vi "pcfs_main_fsm_loop.vi"(8 "error in (no error)":errorcluster, 11 "pcfs in":refnum<class "pcfs.lvclass">) -> (0 "error out":errorcluster, 3 "pcfs out":refnum<class "pcfs.lvclass">)   [LabVIEW 2015, in "pcfs.lvclass"]
uses:
  pcfs.lvclass
  pcfs.lvclass/pcfs.ctl
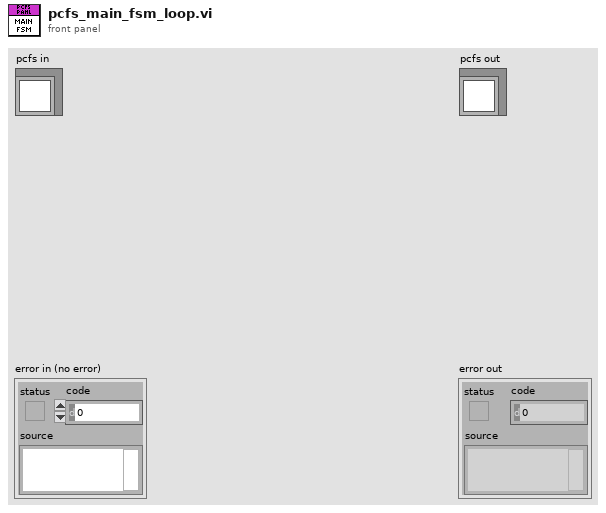
[diagram p1: front panel]
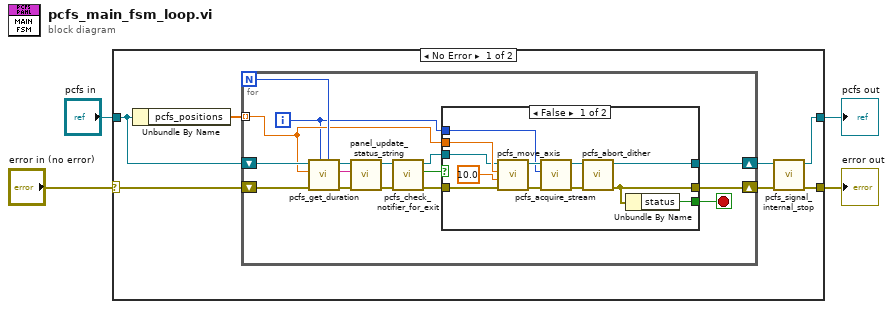
[diagram p0: block diagram]
diagram:
  n1 = case shown="No Error" "error in (no error)" {
    selector: "error in (no error)" -> [w9 w44]
    tunnel: [w7 w44] -> w3
    tunnel: [w5 w43] -> w1
    tunnel: "pcfs in" -> [w10 w43]
    frame No Error {
      n2 = Unbundle By Name(w10) -> ("pcfs_positions"=w11:dbl[])
      n3 = for {
        N -> [w25]
        tunnel: w11 -> [w19] mode=indexing
        shift-right: [w13] -> w6
        shift-left: w10 -> [w27]
        shift-right: [w14] -> w8
        shift-left: w9 -> [w26]
        i -> [w12]
        stop <- w16 stop-if-true
        n4 = call "pcfs_get_duration.vi"("total_steps"=w25, "current_iteration"=w12, "error in (no error)"=w26, "current_position"=w19, "scan_panel in"=w27) -> ("error out"=w24:errorcluster, "time_remaining"=w22:string, "scan_panel out"=w23:refnum<class "pcfs.lvclass">)  [unwired: 4 in]
        n5 = call-dynamic "panel_update_status_string.vi"("error in (no error)"=w24, "String"=w22, "scan_panel in"=w23) -> ("error out"=w21:errorcluster, "scan_panel out"=w20:refnum<class "pcfs.lvclass">)  [unwired: 7 in]
        n6 = call "pcfs_check_notifier_for_exit.vi"("error in (no error)"=w21, "pcfs in"=w20) -> ("error out"=w17:errorcluster, "exit?"=w15:bool, "pcfs out"=w18:refnum<class "pcfs.lvclass">)  [unwired: 7 in]
        n7 = case shown="False" w15 {
          selector: w15 -> [_ w42]
          tunnel: w19 -> [w39 _]
          tunnel: w18 -> [w37 w40]
          tunnel: w17 -> [w36 w41]
          tunnel: [w33 w42] -> w16
          tunnel: [w32 w41] -> w14
          tunnel: [w31 w40] -> w13
          tunnel: w12 -> [w28 _]
          frame False {
            n8 = call "pcfs_move_axis.vi"("error in (no error)"=w36, "Speed"=10.0, "position"=w39, "pcfs in"=w37) -> ("error out"=w30:errorcluster, "pcfs out"=w29:refnum<class "pcfs.lvclass">)  [unwired: 6 in]
            n9 = call "pcfs_acquire_stream.vi"("error in (no error)"=w30, "position_number"=w28, "pcfs in"=w29) -> ("error out"=w35:errorcluster, "pcfs out"=w34:refnum<class "pcfs.lvclass">)  [unwired: 7 in]
            n10 = call "pcfs_abort_dither.vi"("error in (no error)"=w35, "pcfs in"=w34) -> ("error out"=w32:errorcluster, "pcfs out"=w31:refnum<class "pcfs.lvclass">)  [unwired: 8 in]
            n11 = Unbundle By Name(w32) -> ("status"=w33:bool)
          }
          frame True {
          }
        }
      }
      n12 = call "pcfs_signal_internal_stop.vi"("error in (no error)"=w8, "pcfs in"=w6) -> ("error out"=w7:errorcluster, "pcfs out"=w5:refnum<class "pcfs.lvclass">)  [unwired: 8 in]
    }
    frame Error {
    }
  }
  "error out" <- w3
  "pcfs out" <- w1
